vi "test Random Consumer Messages.vi"(8 "error in (no error)":errorcluster, 11 "TestCase in":refnum<class "Multi Consumer Test Case.lvclass">) -> (0 "error out":errorcluster, 3 "TestCase out":refnum<class "Multi Consumer Test Case.lvclass">)   [LabVIEW 2017, in "Multi Consumer Test Case.lvclass"]
uses:
  Multi Consumer Test Case.lvclass
  Support/Messages/Consumer Name Request Message/Consumer Name Request Message.lvclass
  C:/github/niveristand-custom-device-message-library/Source/Message/Abstract Message/Abstract Message.lvclass
  Support/Messages/Consumer Name Response Message/Consumer Name Response Message.lvclass
  Message/Shutdown Message/Shutdown Message.lvclass
  Multi Consumer Test Case.lvclass/Multi Consumer Test Case.ctl
  Support/Messages/Consumer Name Response Message/Consumer Name Response Message.lvclass/Consumer Name Response Message.ctl
  Support/Messages/Consumer Name Response Message/Read Consumer Name.vi
  Producer/Abstract Producer/Abstract Producer.lvclass
  <vilib>/addons/_JKI Toolkits/VI Tester/TestCase.llb/TestCase.lvclass
  C:/Program Files (x86)/National Instruments/LabVIEW 2017/vi.lib/addons/_JKI Toolkits/VI Tester/TestCase.llb/TestCase.lvclass
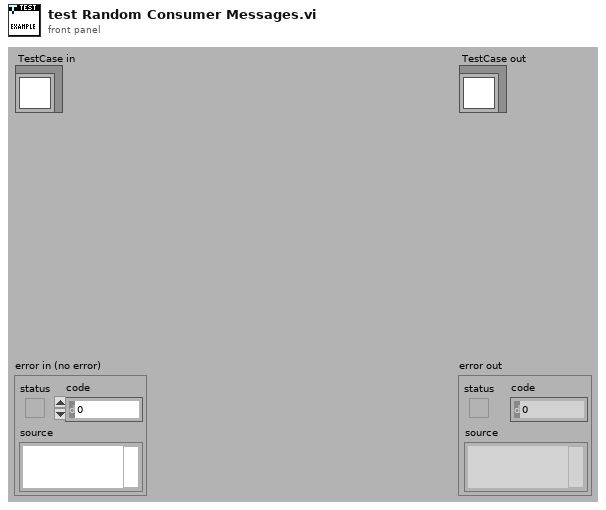
[diagram p1: front panel]
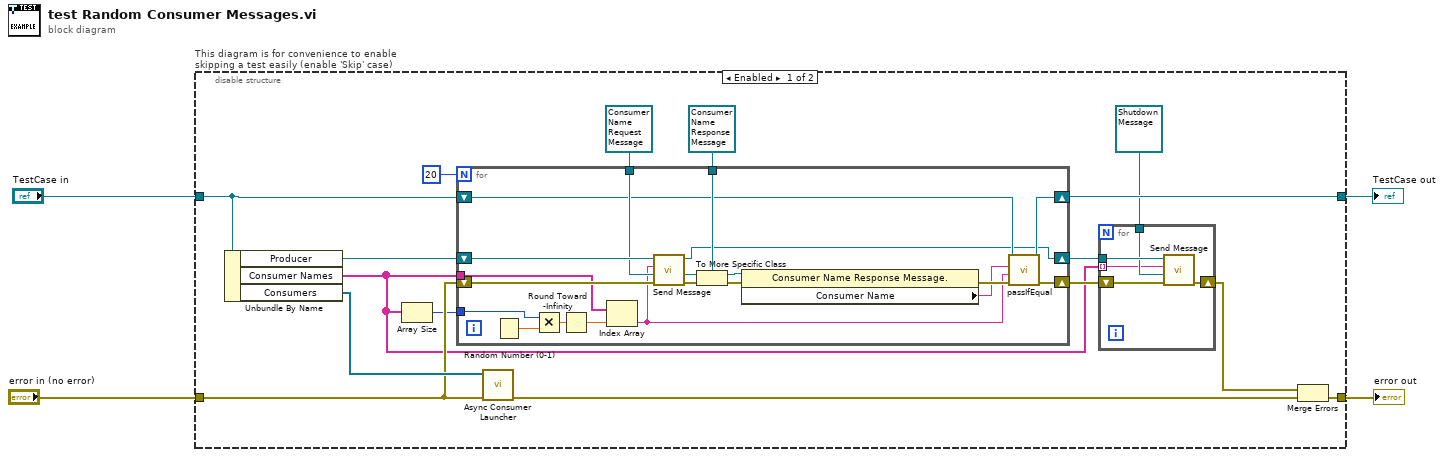
[diagram p0: block diagram]
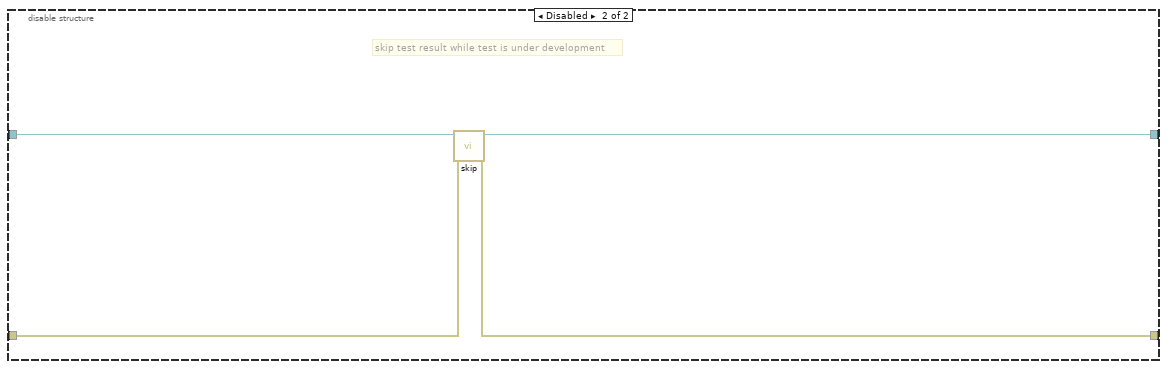
[diagram p2: hidden frame]
diagram:
  n1 = disable-structure "This diagram is for convenience to enable skipping a test easily (enable 'Skip' case)" shown="Enabled" {
    disable-tunnel: "TestCase in" -> [w14 w49]
    disable-tunnel: [w13 w47] -> w1
    disable-tunnel: [w7 w48] -> w3
    disable-tunnel: "error in (no error)" -> [w15 w46]
    frame Enabled {
      n2 = Unbundle By Name(w14) -> ("Producer"=w20:refnum<class "Abstract Producer.lvclass">, "Consumer Names"=w6:string[], "Consumers"=w19:refnum<class "Abstract Consumer.lvclass">[])
      n3 = Array Size(array=w6) -> (size(s)=w5:i32)
      n4 = for {
        N: 20 -> [_]
        tunnel: refnum<class "Consumer Name Request Message.lvclass"> refnum ("Consumer Name Request Message.lvclass") -> [w44]
        tunnel: refnum<class "Consumer Name Response Message.lvclass"> refnum ("Consumer Name Response Message.lvclass") -> [w42]
        tunnel: w6 -> [w36]
        shift-right: [w32] -> w11
        shift-left: w15 -> [w41]
        shift-right: [w30] -> w13
        shift-left: w14 -> [w31]
        shift-right: [w27] -> w10
        shift-left: w20 -> [w45]
        tunnel: w5 -> [w26]
        n5 = Random Number (0-1)() -> (number: 0 to 1=w38:dbl)
        n6 = Multiply(x=w26, y=w38) -> (x*y=w39:dbl)
        n7 = Round Toward -Infinity(1:w39) -> (0:w37:dbl)
        n8 = Index Array(array=w36, index=w37) -> (element=w28:string)
        n9 = call-dynamic "Send Message.vi"("error in (no error)"=w41, "Message in"=w44, "Consumer in"=w28, "Abstract Producer in"=w45) -> ("error out"=w40:errorcluster, "Message out"=w43:refnum<class "Abstract Message.lvclass">, "Abstract Producer out"=w27:refnum<class "Abstract Producer.lvclass">)  [unwired: 5 in]
        n10 = To More Specific Class(target class=w42, reference=w43, error in=w40) -> (specific class reference=w35:refnum<class "Consumer Name Response Message.lvclass">, error out=w34:errorcluster)
        n11 = property class="Consumer Name Response Message."(reference=w35, error in=w34) -> (error out=w33:errorcluster, "Consumer Name"=w29:string)  [unwired: 1 out]
        n12 = call-dynamic "passIfEqual.vi"("error in (no error)"=w33, "y"=w28, "x"=w29, "TestCase in"=w31) -> ("error out"=w32:errorcluster, "TestCase out"=w30:refnum<class "Multi Consumer Test Case.lvclass">)  [unwired: 6 in]
      }
      n13 = call "Async Consumer Launcher.vi"("error in (no error)"=w15, "Consumers"=w19) -> ("error out"=w12:errorcluster)  [unwired: 9 in]
      n14 = for {
        shift-right: [w21] -> w8
        shift-left: w11 -> [w24]
        tunnel: w10 -> [w25]
        tunnel: refnum<class "Shutdown Message.lvclass"> refnum ("Messaging.lvlib:Message.lvlib:Shutdown Message.lvclass") -> [w23]
        tunnel: w6 -> [w22] mode=indexing
        n15 = call-dynamic "Send Message.vi"("error in (no error)"=w24, "Message in"=w23, "Consumer in"=w22, "Abstract Producer in"=w25) -> ("error out"=w21:errorcluster)  [unwired: 5 in, 2 out]
      }
      n16 = Merge Errors(w8, w12) -> (w7:errorcluster)
    }
    frame Disabled {
      # "skip test result while test is under development"
      n17 = call <vilib>:"skip.vi"("error in (no error)"=w46, "TestCase in"=w49) -> ("error out"=w48:errorcluster, "TestCase out"=w47:refnum<class "Multi Consumer Test Case.lvclass">)  [unwired: 8 in]
    }
  }
  "error out" <- w3
  "TestCase out" <- w1
